vi "_intersectStringArrays.vi"(9 "Array2":string[](array[string]), 10 "Array1":string[](array[string])) -> (2 "Union":string[](array[string]))   [LabVIEW 2013, in "tWorkerController.lvlib" / "tWorkerController.lvclass"]
uses:
  tWorkerController.lvclass
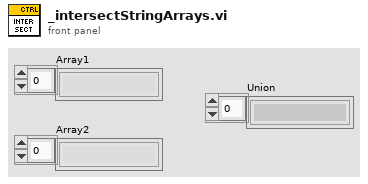
[diagram p1: front panel]
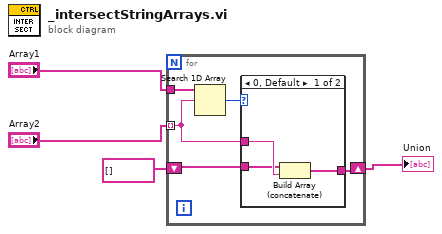
[diagram p0: block diagram]
diagram:
  n1 = for {
    tunnel: "Array2" -> [w7] mode=indexing
    shift-right: [w5] -> w1
    shift-left: string[] [] -> [w6]
    tunnel: "Array1" -> [w9]
    n2 = Search 1D Array(1D array=w9, element=w7) -> (index of element=w8:i32)  [unwired: 1 in]
    n3 = case shown="0, Default" w8 {
      tunnel: w7 -> [w12 _]
      tunnel: w6 -> [w11 w13]
      tunnel: [w10 w13] -> w5
      frame 0, Default {
        n4 = Build Array (concatenate)(w11, w12) -> (w10:string[])
      }
      frame -1 {
      }
    }
  }
  "Union" <- w1
